vi "Exemplo.vi"() -> ()   [LabVIEW 2021]
uses:
  <vilib>/Analysis/3filter.llb/Butterworth Filter (DBL).vi
  <vilib>/measure/NI_MABase.lvlib
  <vilib>/Analysis/NI_AALBase.lvlib
panel:
  out "Tempo de Execução":i64
  out "Gauge":dbl(knob) scale=0.0..1000.0
  out "max value":dbl
  in  "low cutoff freq: fl":dbl=0.12500000000000006 format="%0.4f"
  in  "high cutoff freq: fh":dbl=0.45000000000000007 format="%0.2f"
  out "Waveform Graph 4":dbl[](graph)
  out "Waveform Graph 3":dbl[](graph)
  out "t0":timestamp
  out "Waveform Graph 2":dbl[](graph)
  out "Waveform Graph":dbl[](graph)
  in  "stop":bool
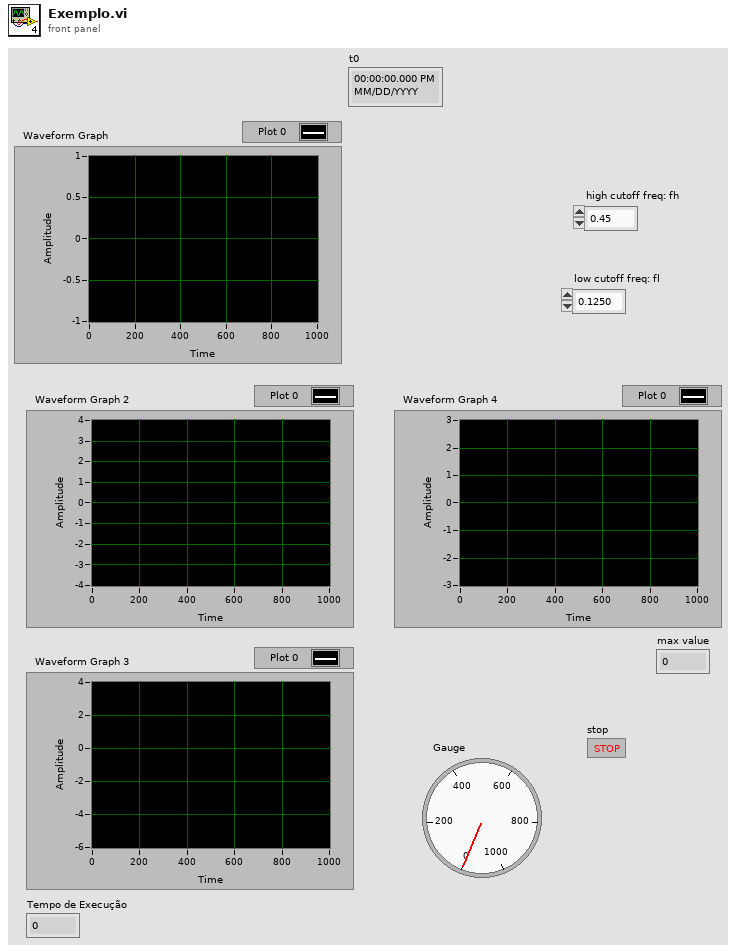
[diagram p1: front panel]
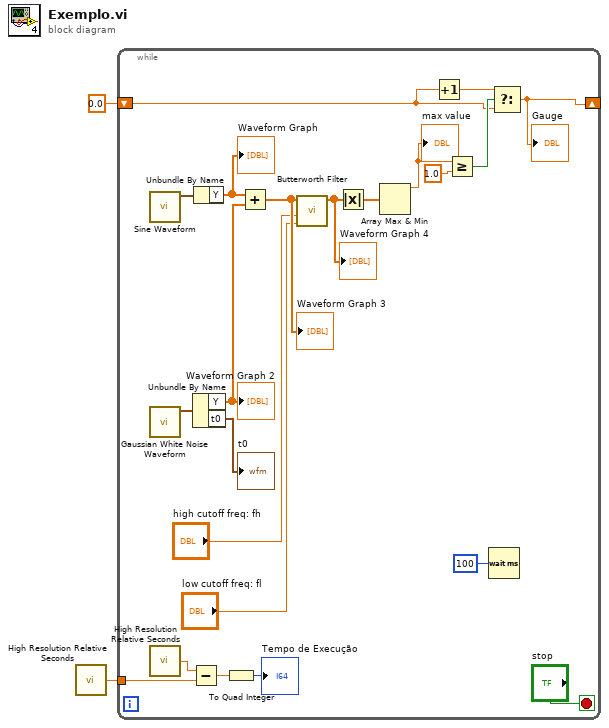
[diagram p0: block diagram]
diagram:
  n1 = call <vilib>:"High Resolution Relative Seconds.vi"() -> ("relative seconds"=w2:dbl)
  n2 = while {
    tunnel: w2 -> [w21]
    shift-right: [w5] -> _
    shift-left: 0.0 -> [w6]
    stop <- "stop" stop-if-true
    n3 = call <vilib>:"Sine Waveform.vi"() -> ("signal out"=w19:waveform(dbl))  [unwired: 10 in, 1 out]
    n4 = call <vilib>:"Gaussian White Noise Waveform.vi"() -> ("signal out"=w18:waveform(dbl))  [unwired: 10 in, 1 out]
    n5 = call <vilib>:"High Resolution Relative Seconds.vi"() -> ("relative seconds"=w22:dbl)
    n6 = Subtract(x=w22, y=w21) -> (x-y=w20:dbl)
    n7 = Unbundle By Name(w18) -> ("Y"=w15:dbl[], "t0"=→"t0":timestamp)
    "Waveform Graph 2" <- w15
    n8 = Unbundle By Name(w19) -> ("Y"=w16:dbl[])
    "Waveform Graph" <- w16
    n9 = To Quad Integer(1:w20) -> (0:→"Tempo de Execução":i64)
    n10 = Add(x=w16, y=w15) -> (x+y=w14:dbl[])
    "Waveform Graph 3" <- w14
    n11 = call-poly <vilib>:"Butterworth Filter.vi"("low cutoff freq: fl"="low cutoff freq: fl", "high cutoff freq: fh"="high cutoff freq: fh", "X"=w14) -> ("Filtered X"=w11:dbl[])  [unwired: 5 in, 1 out]
    "Waveform Graph 4" <- w11
    n12 = Absolute Value(x=w11) -> (abs(x)=w4:dbl[])
    n13 = Array Max & Min(array=w4) -> (max value=w10:dbl)  [unwired: 3 out]
    "max value" <- w10
    n14 = Increment(x=w6) -> (x+1=w7:dbl)
    n15 = Greater Or Equal?(x=w10, y=1.0) -> (x >= y?=w8:bool)
    n16 = Wait (ms)(milliseconds to wait=u32 100) -> ()  [unwired: 1 out]
    n17 = Select(t=w7, s=w8, f=w6) -> (s? t:f=w5:dbl)
    "Gauge" <- w5
  }
